vi "Write Target Integer.vi"(8 "error in (no error)":errorcluster, 10 "Target Integer":u32, 11 "Wait On Integer Step Config in":refnum<class "Wait On Integer Step Config.lvclass">) -> (0 "error out":errorcluster, 3 "Wait On Integer Step Config out":refnum<class "Wait On Integer Step Config.lvclass">)   [LabVIEW 2015, in "Wait On Integer Step Config.lvclass"]
uses:
  Wait On Integer Step Config.lvclass
  Wait On Integer Step Config.lvclass/Wait On Integer Step Config.ctl
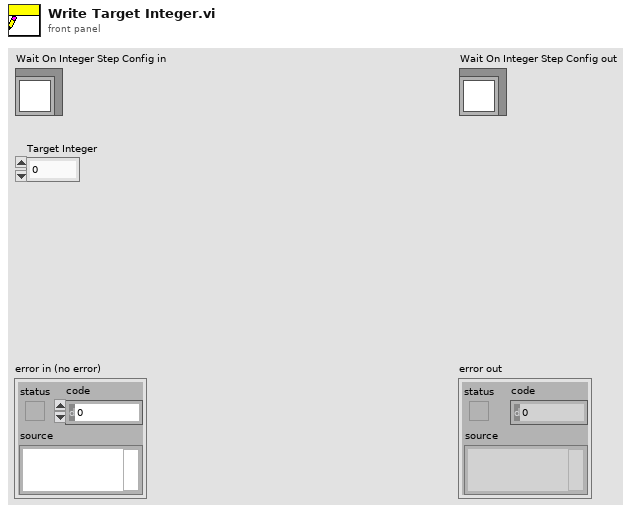
[diagram p1: front panel]
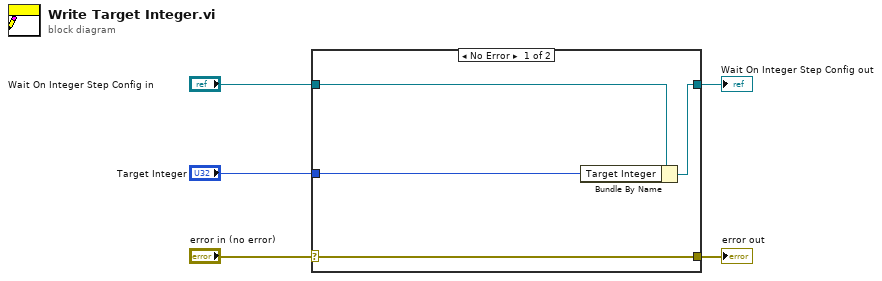
[diagram p0: block diagram]
diagram:
  n1 = case shown="No Error" "error in (no error)" {
    selector: "error in (no error)" -> [w9 w10]
    tunnel: [w9 w10] -> w4
    tunnel: [w7 w11] -> w2
    tunnel: "Wait On Integer Step Config in" -> [w8 w11]
    tunnel: "Target Integer" -> [w6 _]
    frame No Error {
      n2 = Bundle By Name(cluster=w8, "Target Integer"=w6) -> (w7:refnum<class "Wait On Integer Step Config.lvclass">)
    }
    frame Error {
    }
  }
  "error out" <- w4
  "Wait On Integer Step Config out" <- w2
